vi "AH Bridge Setup.vi"(2 "Wait Time (mS)":u32, 3 "Read Frequency":bool, 4 "AH 2500?":bool, 5 "AVE TIME":u32, 6 "Return Dissapation":u8, 7 "Instrument Address":refnum<visa-resource-name>) -> (0 "Error Out":errorcluster, 1 "dup Instrument Address":refnum<visa-resource-name>)   [LabVIEW 2020]
panel:
  out "Commands":string[](array[string])
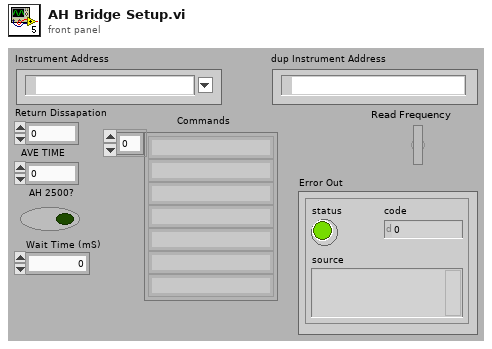
[diagram p1: front panel]
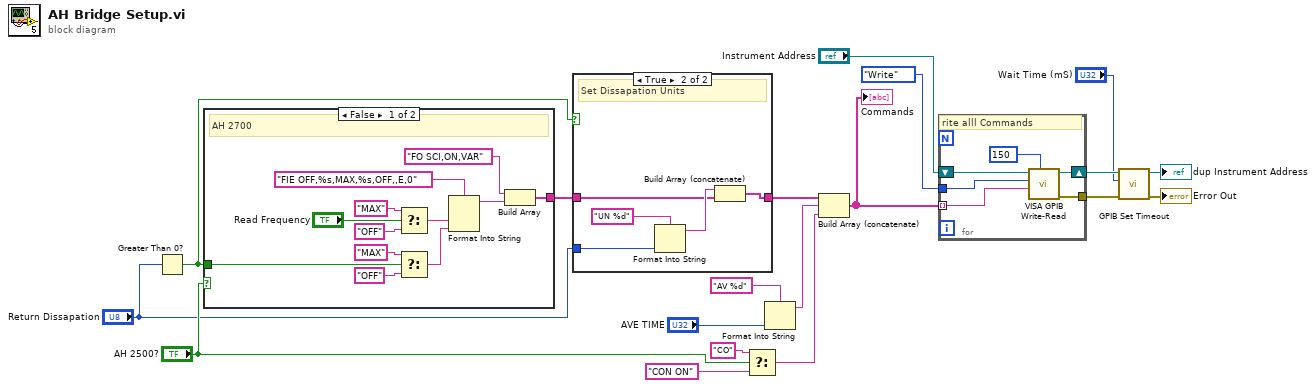
[diagram p0: block diagram]
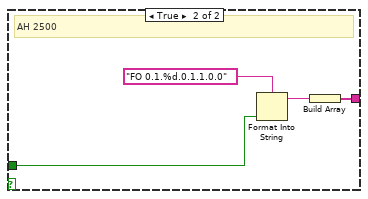
[diagram p2: hidden frame]
diagram:
  n1 = Greater Than 0?(x="Return Dissapation") -> (x > 0?=w1:bool)
  n2 = case shown="False" "AH 2500?" {
    tunnel: [w29 w34] -> w2
    tunnel: w1 -> [w21 w32]
    frame False {
      # "AH 2700"
      n3 = Select(t="MAX", s="Read Frequency", f="OFF") -> (s? t:f=w24:string)
      n4 = Select(t="MAX", s=w21, f="OFF") -> (s? t:f=w22:string)
      n5 = Format Into String(format string="FIE OFF,%s,MAX,%s,OFF,,E,0", w24, w22) -> (resulting string=w28:string)  [unwired: 2 in, 1 out]
      n6 = Build Array("FO SCI,ON,VAR", w28) -> (w29:string[])
    }
    frame True {
      # "AH 2500"
      n7 = Format Into String(format string="FO 0.1.%d.0.1.1.0.0", w32) -> (resulting string=w35:string)  [unwired: 2 in, 1 out]
      n8 = Build Array(w35) -> (w34:string[])
    }
  }
  n9 = case shown="True" w1 {
    tunnel: [w36 w41] -> w5
    tunnel: "Return Dissapation" -> [_ w39]
    tunnel: w2 -> [w36 w37]
    frame False {
      # "No Dissapation"
    }
    frame True {
      # "Set Dissapation Units"
      n10 = Format Into String(format string="UN %d" ("Input String"), w39) -> (resulting string=w38:string)  [unwired: 2 in, 1 out]
      n11 = Build Array (concatenate)(w38, w37) -> (w41:string[])
    }
  }
  n12 = Select(t="CO" ("Command"), s="AH 2500?", f="CON ON") -> (s? t:f=w10:string)
  n13 = Format Into String(format string="AV %d", "AVE TIME") -> (resulting string=w9:string)  [unwired: 2 in, 1 out]
  n14 = Build Array (concatenate)(w5, w9, w10) -> (w6:string[])
  "Commands" <- w6
  n15 = for {
    tunnel: enum16{"Write", "Read", "Write & Read"}."Write" ("Action") -> [w45]
    tunnel: [w43] -> w14
    shift-right: [w44] -> w15
    shift-left: "Instrument Address" -> [w46]
    tunnel: w6 -> [w42] mode=indexing
    # "rite alll Commands"
    n16 = call "VISA GPIB Write-Read.vi"("Wait (ms)"=u32 150 ("wait (mS)"), "Command"=w42, "Action"=w45, "VISA resource name"=w46) -> ("error out"=w43:errorcluster, "dup VISA Session"=w44:refnum<visa-resource-name>)  [unwired: 4 in, 2 out]
  }
  n17 = call "GPIB Set Timeout.vi"("Error In"=w14, "Timeout"="Wait Time (mS)", "VISA resource name"=w15) -> ("Error Out"=→"Error Out":errorcluster, "dup VISA resource name"=→"dup Instrument Address":refnum<visa-resource-name>)  [unwired: 2 in, 1 out]
